vi "PrepareGameState.vi"(8 "error in (no error)":errorcluster, 11 "Game in":refnum<class "Game.lvclass">) -> (0 "error out":errorcluster, 1 "Bot2GameState":T1, 2 "Bot1GameState":T1, 3 "Game out":refnum<class "Game.lvclass">)   [LabVIEW 2015, in "TronviewGame.lvlib" / "Game.lvclass"]
uses:
  Game.lvclass
  TronVIEWBotAPI/GameState.ctl
  Board/Position.ctl
  Game.lvclass/Game.ctl
  Player/Player.lvclass/Player.ctl
  Board/Board.lvclass/Board.ctl
  Board/GetOccupancyBoard.vi
  Board/GetPlayer1Position.vi
  Board/GetPlayer2Position.vi
  Player/GetPlayerName.vi
  Board/FindFieldPosition.vi
  Board/Board.lvclass
  TronVIEWBotAPI/TronVIEWBotAPI.lvlib
  Player/Player.lvclass
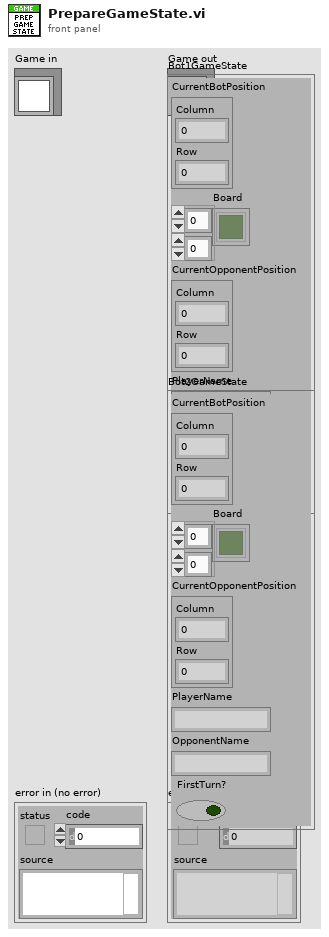
[diagram p1: front panel]
types:
  T1 = typedef "TronVIEWBotAPI.lvlib/GameState.ctl" = cluster{"CurrentBotPosition":T2, "Board":bool[][], "CurrentOpponentPosition":T2, "PlayerName":string, "OpponentName":string, "FirstTurn?":bool}
  T2 = typedef "TronviewGame.lvlib/Board.lvclass/Position.ctl" = cluster{"Column":i32, "Row":i32}
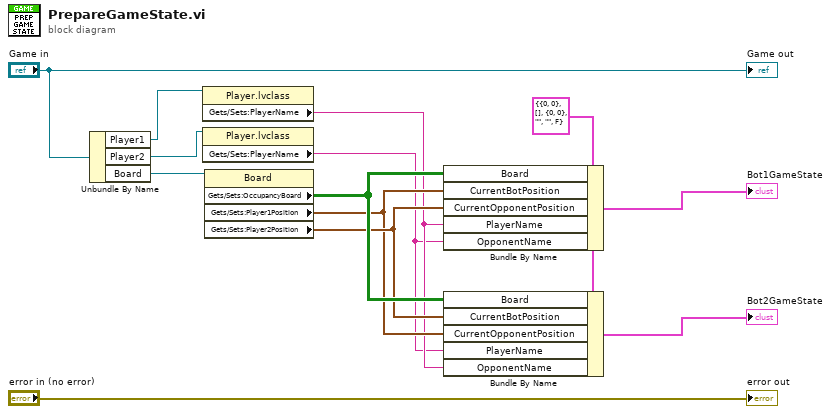
[diagram p0: block diagram]
diagram:
  w10 = T1 {"CurrentBotPosition"={"Column"=0, "Row"=0}, "Board"=[], "CurrentOpponentPosition"={"Column"=0, "Row"=0}, "PlayerName"="", "OpponentName"="", "FirstTurn?"=FALSE} ("GameState")
  n1 = Unbundle By Name("Game in") -> ("Player1"=w4:refnum<class "Player.lvclass">, "Player2"=w3:refnum<class "Player.lvclass">, "Board"=w11:refnum<class "Board.lvclass">)
  n2 = property class="Player.lvclass"(reference=w4) -> ("Gets/Sets:PlayerName"=w2:string)  [unwired: 1 in, 2 out]
  n3 = property class="Player.lvclass"(reference=w3) -> ("Gets/Sets:PlayerName"=w1:string)  [unwired: 1 in, 2 out]
  n4 = property class="Board"(reference=w11) -> ("Gets/Sets:OccupancyBoard"=w7:bool[][], "Gets/Sets:Player1Position"=w5:T2, "Gets/Sets:Player2Position"=w6:T2)  [unwired: 1 in, 2 out]
  n5 = Bundle By Name(cluster=w10, "Board"=w7, "CurrentBotPosition"=w5, "CurrentOpponentPosition"=w6, "PlayerName"=w2, "OpponentName"=w1) -> (→"Bot1GameState":T1)
  n6 = Bundle By Name(cluster=w10, "Board"=w7, "CurrentBotPosition"=w6, "CurrentOpponentPosition"=w5, "PlayerName"=w1, "OpponentName"=w2) -> (→"Bot2GameState":T1)
  "error out" <- "error in (no error)"
  "Game out" <- "Game in"
